vi "create.vi"(5 "subresults":refnum<class "result.lvclass">[](array[class]), 9 "error":errorcluster, 10 "data":variant, 11 "data ID":string) -> (3 "result out":refnum<class "result.lvclass">)   [LabVIEW 2015, in "result.lvclass"]
uses:
  result.lvclass
  result.lvclass/result.ctl
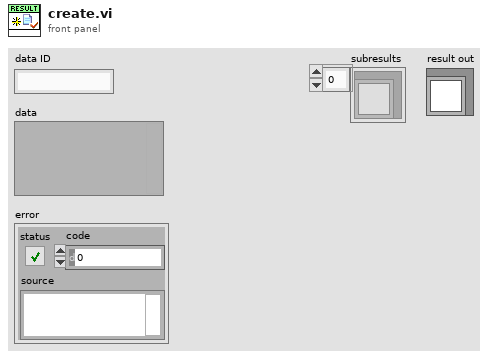
[diagram p1: front panel]
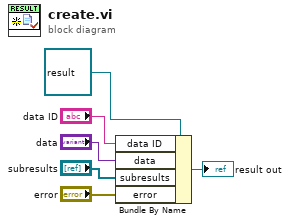
[diagram p0: block diagram]
diagram:
  n1 = Bundle By Name(cluster=refnum<class "result.lvclass"> refnum ("result in"), "data ID"="data ID", "data"="data", "subresults"="subresults", "error"="error") -> (→"result out":refnum<class "result.lvclass">)
